vi "Pre Launch Init.vi"(11 "JoyStick in":refnum<class "JoyStick.lvclass"> caption="操作者输入") -> (0 "error out":errorcluster caption="错误输出", 3 "JoyStick out":refnum<class "JoyStick.lvclass"> caption="操作者输出")   [LabVIEW 2014, in "JoyStick.lvlib" / "JoyStick.lvclass"]
doc: "(<B>Filename</B>: Actor Framework.lvlib:Actor.lvclass:Pre Launch Init.vi)\n\nDefines behavior that occurs after the Launch Nested Actor method is invoked but before the actor's Actor Core method begins running.\n\nBy default, this method does nothing. A descendant class may override it to define behavior."
uses:
  JoyStick.lvclass
  Wrapper_lib/zsActor/ActorWrapper.lvclass
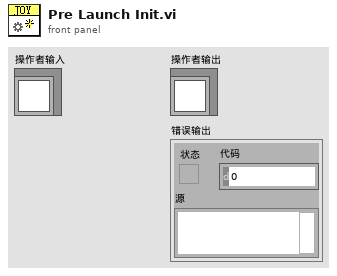
[diagram p1: front panel]
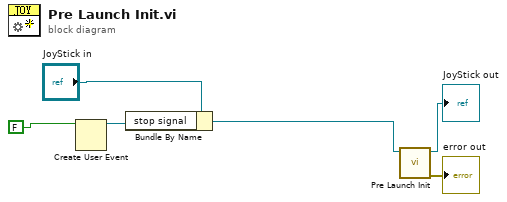
[diagram p0: block diagram]
diagram:
  n1 = Create User Event(user event datatype=FALSE ("stop signal")) -> (user event=w3:refnum<user-event>)  [unwired: 1 in, 1 out]
  n2 = Bundle By Name(cluster="JoyStick in", "stop signal"=w3) -> (w1:refnum<class "JoyStick.lvclass">)
  n3 = call-parent "Pre Launch Init.vi"("Actor in"=w1) -> ("error out"=→"error out":errorcluster, "Actor out"=→"JoyStick out":refnum<class "JoyStick.lvclass">)  [unwired: 9 in]
